vi "InitializeCurveList.vi"(10 "循环树形":refnum<vi>, 11 "ListBox输入":refnum<vi>) -> (0 "符号数组":picture[](array[picture]), 1 "颜色符号列表":cluster{"项名":string, "颜色":u32, "符号":i32}[](array[cluster]), 2 "Tree引用输出":refnum<vi>, 3 "List引用输出":refnum<vi>)   [LabVIEW 2020, in "Curve Editor.lvlib"]
uses:
  Curve Editor.lvlib
panel:
  # "给动作列表添加项目及符号集合，并给树形列表添加符号集合，并返回符号集合"
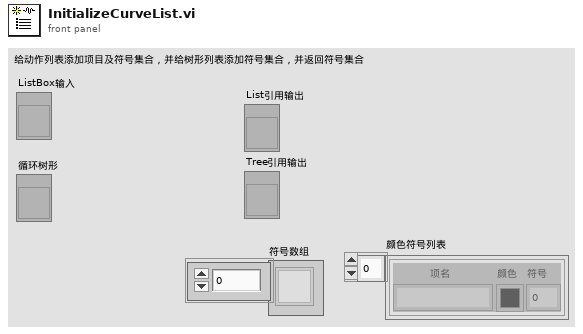
[diagram p1: front panel]
types:
  T1 = typedef "imagedata.ctl" = cluster{"image type":i32, "image depth":i32, "image":u8[], "mask":u8[], "colors":u32[], "Rectangle":cluster{"left":i16, "top":i16, "right":i16, "bottom":i16}}
  T2 = cluster{"image type":i32, "image depth":i32, "image":u8[], "mask":u8[], "colors":u32[], "Rectangle":cluster{"left":i16, "top":i16, "right":i16, "bottom":i16}}[]
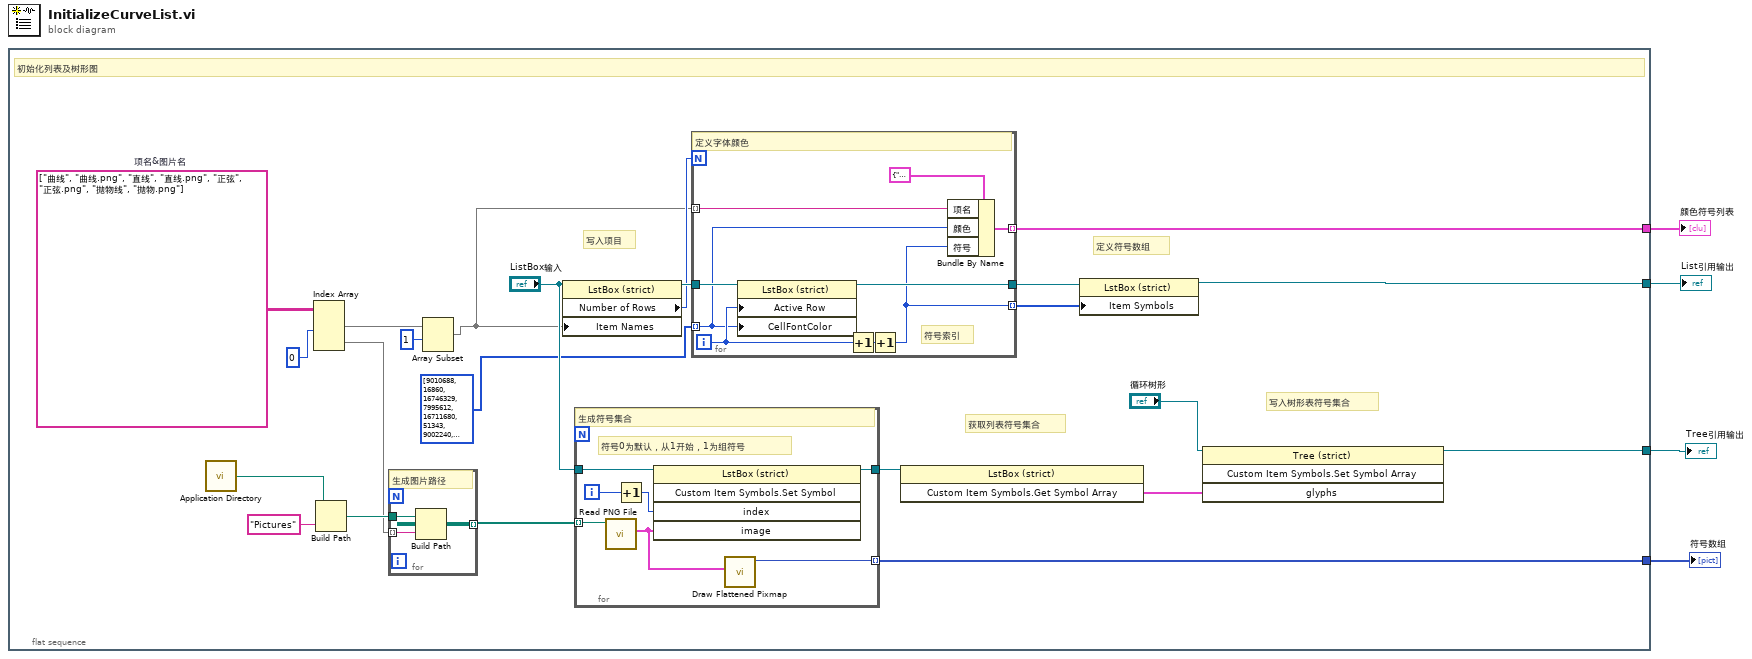
[diagram p0: block diagram]
diagram:
  n1 = flat-sequence {
    tunnel: [w10] -> w4
    tunnel: [w9] -> w3
    tunnel: [w7] -> w2
    tunnel: [w6] -> w1
    frame #0 {
      w17 = string[][] [["曲线", "曲线.png"], ["直线", "直线.png"], ["正弦", "正弦.png"], ["抛物线", "抛物.png"]]  # 项名&图片名
      # "写入树形表符号集合"
      # "获取列表符号集合"
      # "定义符号数组"
      # "写入项目"
      # "初始化列表及树形图"
      n2 = call <vilib>:"Application Directory.vi"() -> ("Application Directory"=w21:path)
      n3 = Index Array(array=w17, index (col) #1=0) -> (element #1=w12:string[], element #2=w15:string[])  [unwired: 3 in]
      n4 = Build Path(base path=w21, name or relative path="Pictures" ("名称或相对路径")) -> (appended path=w19:path)
      n5 = for {
        tunnel: w19 -> [w30]
        tunnel: [w29] -> w18 mode=indexing
        tunnel: w15 -> [w28] mode=indexing
        # "生成图片路径"
        n6 = Build Path(base path=w30, name or relative path=w28) -> (appended path=w29:path)
      }
      n7 = Array Subset(array=w12, index=1 ("索引")) -> (w5:string[])  [unwired: 1 in]
      n8 = property class="LstBox (strict)"(reference="ListBox输入", "Item Names"=w5) -> (reference out=w23:refnum<vi>, "Number of Rows"=w22:u32)  [unwired: 1 in, 1 out]
      n9 = for {
        tunnel: "ListBox输入" -> [w37]
        tunnel: w18 -> [w36] mode=indexing
        tunnel: [w33] -> w7 mode=indexing
        tunnel: [w31] -> w26
        i -> [w35]
        # "符号0为默认，从1开始，1为组符号"
        # "生成符号集合"
        n10 = call <vilib>:"Read PNG File.vi"("path to PNG file"=w36) -> ("image data"=w34:T1)  [unwired: 8 in, 2 out]
        n11 = Increment(x=w35) -> (x+1=w32:i32)
        n12 = invoke class="LstBox (strict)" method="Custom Item Symbols.Set Symbol"(reference=w37, "index"=w32, "image"=w34) -> (reference out=w31:refnum<vi>)  [unwired: 2 in, 4 out]
        n13 = call <vilib>:"Draw Flattened Pixmap.vi"("image data"=w34) -> ("new picture"=w33:picture)  [unwired: 8 in]
      }
      n14 = for {
        N: w22 -> [_]
        tunnel: w23 -> [w46]
        tunnel: u32[] [9010688, 16860, 16746329, 7995612, 16711680, 51343, 9002240, 29469, 180, 56063, 0, 0, 0, 0, 0] -> [w39] mode=indexing
        tunnel: [w45] -> w14
        tunnel: [w40] -> w13 mode=indexing
        tunnel: [w41] -> w6 mode=indexing
        tunnel: w5 -> [w38] mode=indexing
        i -> [w44]
        # "符号索引"
        # "定义字体颜色"
        n15 = property class="LstBox (strict)"(reference=w46, "Active Row"=w44, "CellFontColor"=w39) -> (reference out=w45:refnum<vi>)  [unwired: 1 in, 1 out]
        n16 = Increment(x=w44) -> (x+1=w43:i32)
        n17 = Increment(x=w43) -> (x+1=w40:i32)
        n18 = Bundle By Name(cluster=cluster{"项名":string, "颜色":u32, "符号":i32} {"项名"="", "颜色"=0, "符号"=0} ("簇"), "项名"=w38, "颜色"=w39, "符号"=w40) -> (w41:cluster{"项名":string, "颜色":u32, "符号":i32})
      }
      n19 = invoke class="LstBox (strict)" method="Custom Item Symbols.Get Symbol Array"(reference=w26) -> ("Custom Item Symbols:Get Symbol Array"=w27:T2)  [unwired: 2 in, 2 out]
      n20 = property class="LstBox (strict)"(reference=w14, "Item Symbols"=w13) -> (reference out=w10:refnum<vi>)  [unwired: 1 in, 1 out]
      n21 = invoke class="Tree (strict)" method="Custom Item Symbols.Set Symbol Array"(reference="循环树形", "glyphs"=w27) -> (reference out=w9:refnum<vi>)  [unwired: 2 in, 3 out]
    }
  }
  "List引用输出" <- w4
  "Tree引用输出" <- w3
  "符号数组" <- w2
  "颜色符号列表" <- w1
